vi "GUI_HV.vi"() -> ()   [LabVIEW 2013]
uses:
  shared programs/GUI_Template/GUI_master/tcp_new_data_event.ctl
  shared programs/GUI_Template/GUI_master/tcp new data cluster.ctl
panel:
  in  "value::1":dbl=0.5 caption="kV" min=-25.0 max=25.0 format="%_4f"
  in  "stop":bool
  out "tcp data event":T1
  out "error IO 2":errorcluster
  in  "GUIdevice 1":string="TS-HV"
  # "High Voltage"
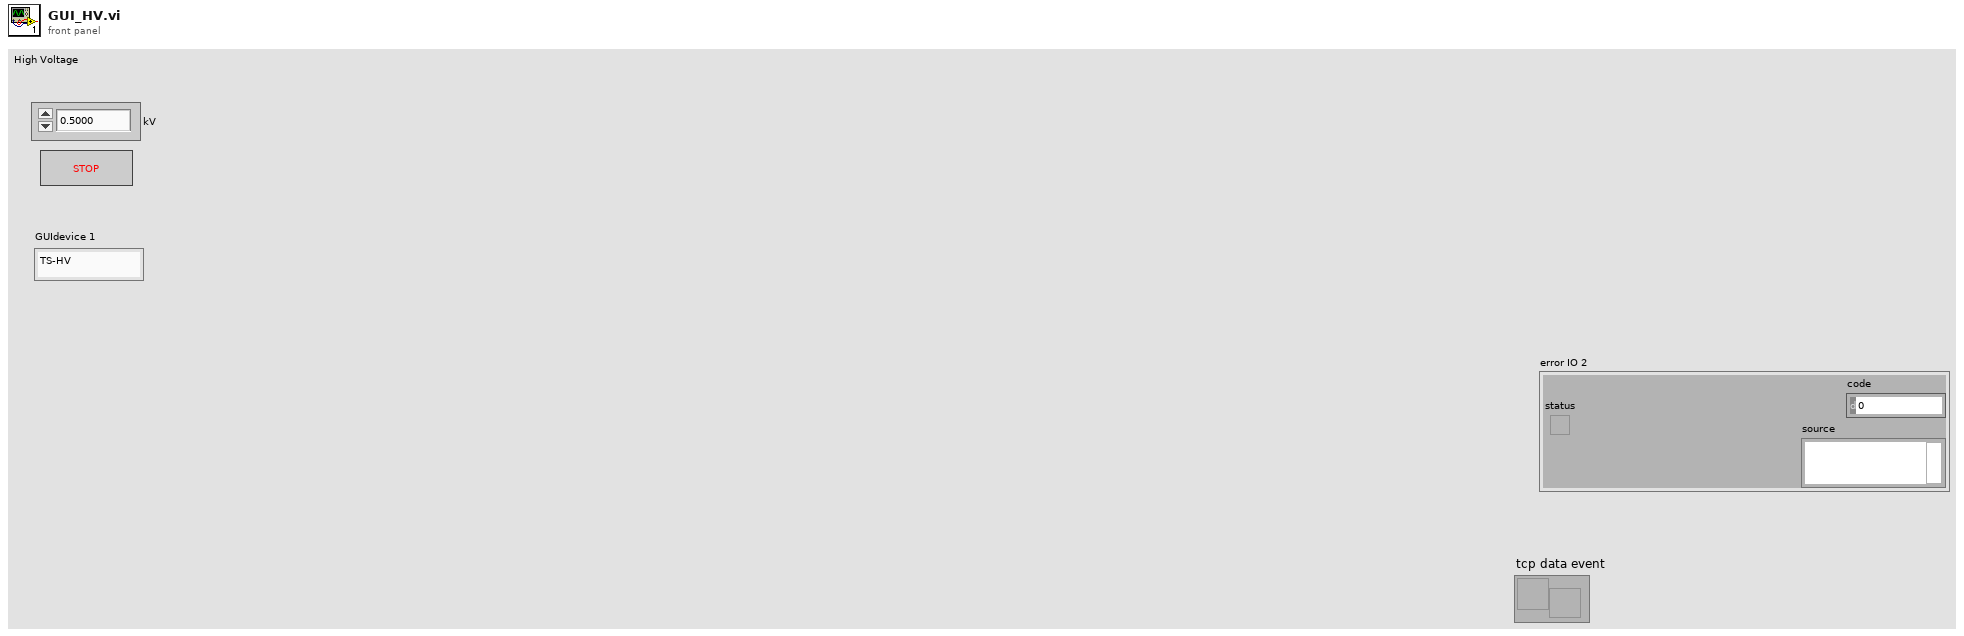
[diagram p1: front panel]
types:
  T1 = typedef "tcp_new_data_event.ctl" = refnum<user-event>
  T2 = typedef "tcp new data cluster.ctl" = cluster{"EventEnum":enum16{"new data", "connection status update"}, "Device name":string}
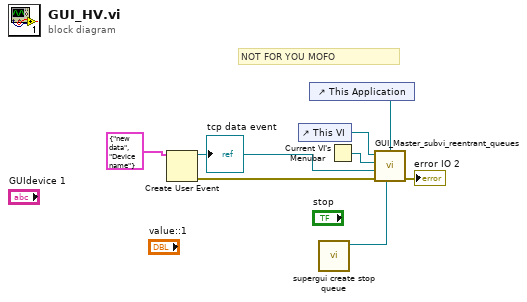
[diagram p0: block diagram]
diagram:
  # "NOT FOR YOU MOFO"
  n1 = Create User Event(user event datatype=T2 {"EventEnum"=enum."new data", "Device name"="Device name"} ("New Event")) -> (user event=w3:refnum<user-event>, error out=w8:errorcluster)  [unwired: 1 in]
  "tcp data event" <- w3
  n2 = control-ref of="This VI"() -> (w5:refnum<vi>)
  n3 = control-ref of="This Application"() -> (w2:refnum<vi>)
  n4 = call "supergui create stop queue.vi"() -> ("STOP Queue out"=w1:refnum<queue>)  [unwired: 11 in]
  n5 = Current VI's Menubar() -> (w6:refnum<k9>)
  n6 = call "GUI_Master_subvi_reentrant_queues.vi"("STOP Queue in"=w1, "This Application"=w2, "error in (no error)"=w8, "tcp data event"=w3, "Caller menu reference"=w6, "Caller VI ref"=w5) -> ("error out"=→"error IO 2":errorcluster)  [unwired: 5 in]
